vi "IPS IL test.vi"() -> ()   [LabVIEW 2013, in "Mercury iXX.lvlib"]
uses:
  Mercury iXX.lvlib
  Public/Controls/Comms Transport Layer.ctl
  Public/Controls/Serial Settings.ctl
  Public/Controls/ISOBus Address.ctl
panel:
  out "Device Details":T1
  in  "Interval between messages (ms)":i16=100
  out "Mode":string
  out "Status":string
  out "Environment_data":T2 {"Nitrogen Level (%)" format="%_4f"; "Helium Level (%)" format="%_4f"; "Temperature (K)" format="%_4f"}
  out "Mag_data":T3 {"Output Voltage (V)" format="%.4f"; "Magnet Current (A)" format="%.4g"; "Output Current (A)" format="%.4g"}
  out "SW HTR\nCONFIRM":bool
  in  "SWITCH\nHEATER":bool
  in  "Magnet Controls":T4
  in  "Ramp Controls":T5 {"Target Rate (T/min)" format="%_5g"; "Target Field (T)" format="%_5g"; "Target Rate (A/min)" format="%_5g"; "Target Current (A)" format="%_5g"}
  out "error out":errorcluster
  in  "stop":bool
  in  "Connection Details":T9={"VISA resource name"="", "Comms Layer"=enum."Ethernet TCP/IP", "IP Address"="", "Serial Configuration"={"Baud Rate"=115200, "Parity"=0, "Data Bits"=8, "Stop Bits"=10, "Flow Control"=0}, "ISOBUS address"=-1} {"Serial Configuration"."Flow Control" items=["None", "XON/XOFF", "RTS/CTS", "XON/XOFF & RTS/CTS", "DTR/DSR", "XON/XOFF & DTR/DSR"]; "Serial Configuration"."Stop Bits" items=["1.0"=10, "2.0"=20]; "Serial Configuration"."Data Bits" items=["7"=7, "8"=8]; "Serial Configuration"."Parity" items=["None", "Odd", "Even"]; "Serial Configuration"."Baud Rate" items=["300"=300, "600"=600, "1200"=1200, "2400"=2400, "4800"=4800, "9600"=9600, "14400"=14400, "19200"=19200, "38400"=38400, "57600"=57600, "115200"=115200]}
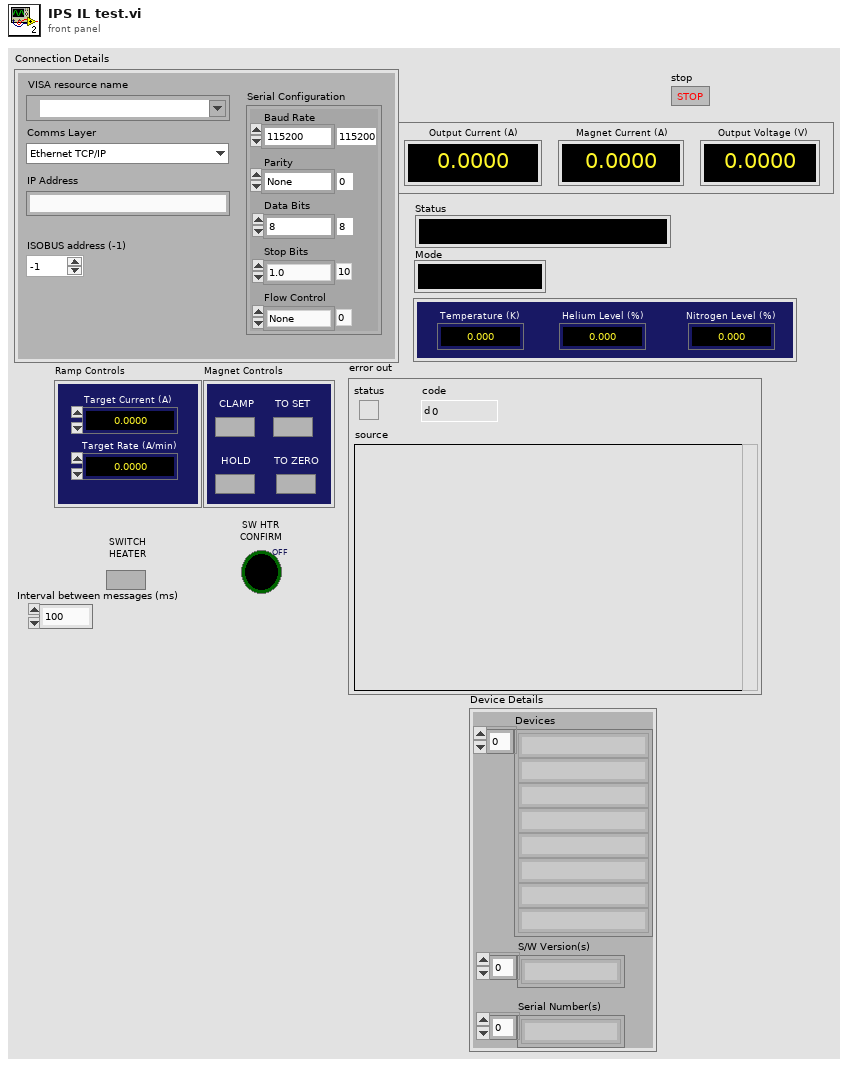
[diagram p1: front panel]
types:
  T1 = cluster{"Devices":string[], "S/W Version(s)":string[], "Serial Number(s)":string[]}
  T2 = cluster{"Temperature (K)":dbl, "Helium Level (%)":dbl, "Nitrogen Level (%)":dbl}
  T3 = cluster{"Output Current (A)":dbl, "Magnet Current (A)":dbl, "Output Voltage (V)":dbl}
  T4 = cluster{"CLAMP":bool, "HOLD":bool, "TO SET":bool, "TO ZERO":bool}
  T5 = cluster{"Target Current (A)":dbl, "Target Rate (A/min)":dbl, "Target Field (T)":dbl, "Target Rate (T/min)":dbl}
  T6 = typedef "Mercury iXX.lvlib/Comms Transport Layer.ctl" = enum16{"Ethernet TCP/IP", "USB", "ISOBus - RS-232", "GPIB"}
  T7 = typedef "Mercury iXX.lvlib/Serial Settings.ctl" = cluster{"Baud Rate":u32, "Parity":u16, "Data Bits":u16, "Stop Bits":u16, "Flow Control":u16}
  T8 = typedef "Mercury iXX.lvlib/ISOBus Address.ctl" = i32
  T9 = cluster{"VISA resource name":refnum<visa-resource-name>, "Comms Layer":T6, "IP Address":string, "Serial Configuration":T7, "ISOBUS address":T8}
  T10 = typedef "Mercury iXX.lvlib/Mercury Reference.ctl" = cluster{"Comms":refnum<visa-resource-name>, "Device ID":string[], "Comms Layer":T6, "Command":string, "Query reference":T11}
  T11 = typedef "Mercury iXX.lvlib/Query Dynamic Reference.ctl" = refnum<vi>
  T12 = cluster{"Current/Field (A/T)":dbl, "Meter_V_Lim":dbl, "Meter_I_lim":dbl}
  T13 = enum16{"Monitor", "Hold", "Clamp", "To Set", "To Zero", "Switch Heater", "Set Points"}
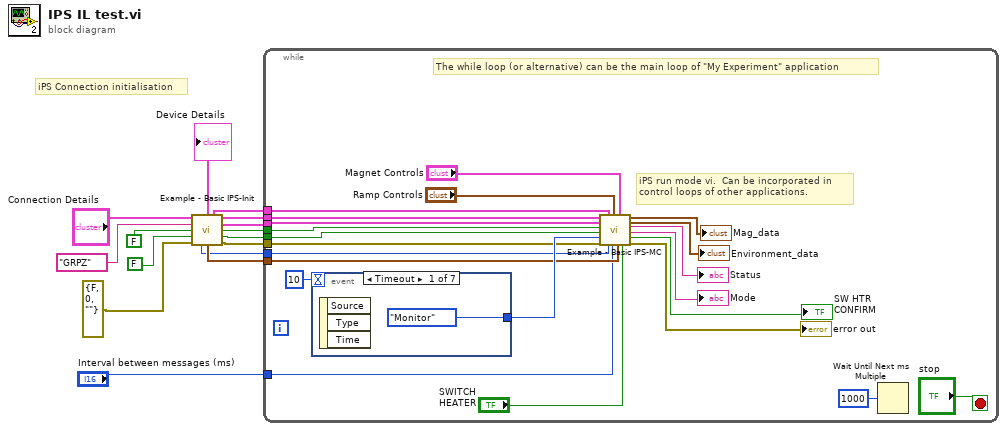
[diagram p0: block diagram]
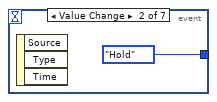
[diagram p2: hidden frame]
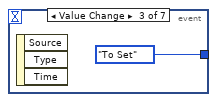
[diagram p3: hidden frame]
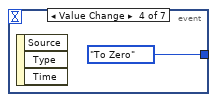
[diagram p4: hidden frame]
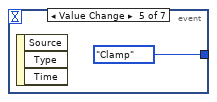
[diagram p5: hidden frame]
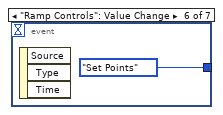
[diagram p6: hidden frame]
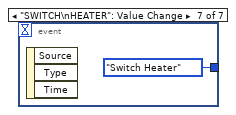
[diagram p7: hidden frame]
diagram:
  # "iPS Connection initialisation"
  n1 = call "Example - Basic IPS-Init.vi"("Connection Details"="Connection Details", "Axis Group"="GRPZ", "ID Query (True)"=FALSE, "Clear Previous Connections (False)"=FALSE, "error in (no error)"=errorcluster {"status"=FALSE, "code"=0, "source"=""}) -> ("Device Details"=→"Device Details":T1, "Merc_Ref_LVL"=w5:T10, "Merc_Ref_Mag"=w10:T10, "Merc_Ref_MB1.T1"=w9:T10, "Temp_Present?"=w8:bool, "LVL_Present?"=w7:bool, "ISOBUS address"=w3:T8, "Range_Data"=w4:T12, "error out"=w6:errorcluster)  [unwired: 1 in, 1 out]
  n2 = while {
    tunnel: w10 -> [w30]
    tunnel: w9 -> [w29]
    tunnel: w8 -> [w28]
    tunnel: w7 -> [w27]
    tunnel: w6 -> [w26]
    tunnel: w5 -> [w22]
    tunnel: w4 -> [w25]
    tunnel: w3 -> [w24]
    tunnel: "Interval between messages (ms)" -> [w23]
    stop <- "stop" stop-if-true
    # "iPS run mode vi.  Can be incorporated in\ncontrol loops of other applications."
    # "The while loop (or alternative) can be the main loop of \"My Experiment\" application"
    n3 = event shown="[0] Timeout" {
      selector: _ -> [_ _ _ _ _ _ _]
      dyn-events: _ -> [_ _ _ _ _ _ _]
      timeout: 10 -> [_ _ _ _ _ _ _]
      tunnel: [T13."Monitor" ("Action") T13."Hold" ("Action") T13."To Set" ("Action") T13."To Zero" ("Action") T13."Clamp" ("Action") T13."Set Points" ("Action") T13."Switch Heater" ("Action")] -> w32
      event Timeout {
        n4 = event-data() -> ()  [unwired: 1 in, 3 out]
      }
      event "Magnet Controls.HOLD": Value Change {
        n5 = event-data() -> ()  [unwired: 1 in, 3 out]
      }
      event "Magnet Controls.TO SET": Value Change {
        n6 = event-data() -> ()  [unwired: 1 in, 3 out]
      }
      event "Magnet Controls.TO ZERO": Value Change {
        n7 = event-data() -> ()  [unwired: 1 in, 3 out]
      }
      event "Magnet Controls.CLAMP": Value Change {
        n8 = event-data() -> ()  [unwired: 1 in, 3 out]
      }
      event "Ramp Controls": Value Change {
        n9 = event-data() -> ()  [unwired: 1 in, 3 out]
      }
      event "SWITCH\nHEATER": Value Change {
        n10 = event-data() -> ()  [unwired: 1 in, 3 out]
      }
    }
    n11 = call "Example - Basic IPS-MC.vi"("Mag_Ref"=w30, "MB1.T1_Ref"=w29, "Temp_present?"=w28, "LVL_present?"=w27, "Action"=w32, "error in (no error)"=w26, "LVL_Ref"=w22, "ISOBUS address"=w24, "Ramp Controls"="Ramp Controls", "Interval between messages (ms)"=w23, "Magnet Controls"="Magnet Controls", "Range data"=w25, "SWITCH\nHEATER"="SWITCH\nHEATER") -> ("Mag_data"=→"Mag_data":T3, "Environment_data"=→"Environment_data":T2, "Status"=→"Status":string, "Mode"=→"Mode":string, "SW HTR\nCONFIRM"=→"SW HTR\nCONFIRM":bool, "error out"=→"error out":errorcluster)  [unwired: 1 in]
    n12 = Wait Until Next ms Multiple(millisecond multiple=u32 1000) -> ()  [unwired: 1 out]
  }
